vi "NI6071E.evt call Read DAQ.vi"(0 "i ref in":refnum<vi>, 2 "Client":string, 3 "Client timeout (10000)":i32=10000, 4 "NI6071E Read":T1={"time limit in sec (-1:auto calculate)"=1.0, "number of scans to read (-1:all)"=1} {"time limit in sec (-1:auto calculate)" format="%0.2f"}, 5 "error in (no error)":errorcluster) -> (14 "i ref out":refnum<vi>, 16 "error unpacking data":bool, 17 "Data":waveform(dbl)[](array[waveform]), 19 "error out":errorcluster)   [LabVIEW 2014, in "NI6071E.lvlib"]
doc: "This VI asks for an event by a synchronous call"
uses:
  NI6071E.lvlib
  NI6071ECommand.ctl
  NI6071ERead.ctl
  CSCore/CSSystem/CoreLib/CoreLib.string 2 byte array.vi
  CSCore/CSSystem/CoreLib/CoreLib.int 2 byte array.vi
  CSCore/CSSystem/CoreLib/CoreLib.byte array 2 string.vi
  CSCore/BaseProcess/BaseProcess.lvlib
  CSCore/CSSystem/CoreLib/CoreLib.lvlib
panel:
  in  "PreAmp Data 2":waveform(dbl)[](graph) caption="Measurement data"
  in  "NI6071E Command":T2=enum."ReadData"
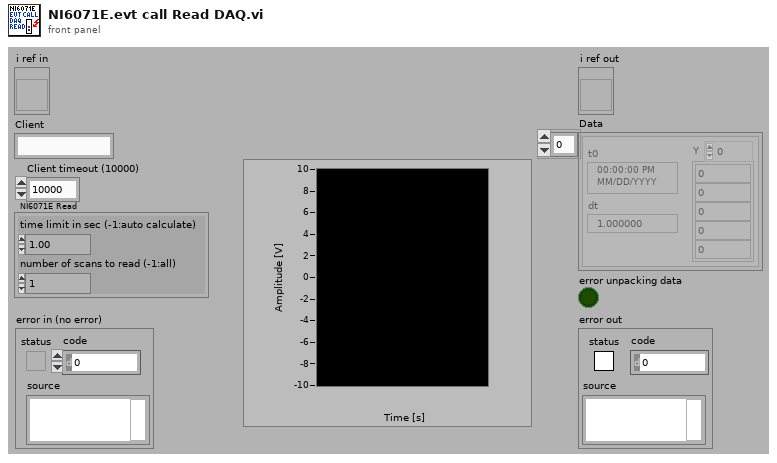
[diagram p1: front panel]
types:
  T1 = typedef "NI6071E.lvlib/NI6071ERead.ctl" = cluster{"time limit in sec (-1:auto calculate)":sgl, "number of scans to read (-1:all)":i32}
  T2 = typedef "NI6071E.lvlib/NI6071ECommand.ctl" = enum16{"Ping", "Reset", "ConfigureDAQ", "StartDAQ", "StopDAQ", "GetDAQStatus", "ReadData", "SaveData", "CloseConnection"}
  T3 = enum16{"simple", "synchronous", "asynchronous", "notification"}
  T4 = typedef "CoreDefs.rawDataType.ctl" = i8[]
  T5 = typedef "CoreDefs.call_type.ctl" = cluster{"Object":string, "Selector":string, "CallType":enum16{"simple", "synchronous", "asynchronous"}, "Async Object":string, "Async Selector":string, "Data Descriptor":T6, "Data":T4, "Error #":i32, "Expire":u32}
  T6 = typedef "BaseProcess.lvlib/BaseProcess.descriptor string definition.ctl" = string
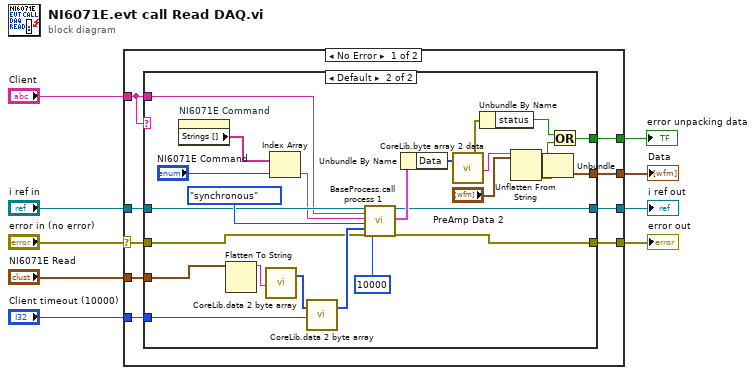
[diagram p0: block diagram]
diagram:
  n1 = case shown="No Error" "error in (no error)" {
    selector: "error in (no error)" -> [w11 w46]
    tunnel: [w18 w46] -> w9
    tunnel: "i ref in" -> [w17 w47]
    tunnel: "Client" -> [w10 _]
    tunnel: [w16 w47] -> w6
    tunnel: "NI6071E Read" -> [w15 _]
    tunnel: [w14 _] -> w4
    tunnel: [w13 _] -> w3
    tunnel: "Client timeout (10000)" -> [w12 _]
    frame No Error {
      n2 = case shown="Default" w10 {
        tunnel: [w19 w44] -> w18
        tunnel: w17 -> [w20 w42]
        tunnel: w10 -> [_ w41]
        tunnel: [w20 w39] -> w16
        tunnel: w15 -> [_ w35]
        tunnel: [_ w33] -> w14
        tunnel: [_ w31] -> w13
        tunnel: w12 -> [_ w23]
        tunnel: w11 -> [w19 w22]
        frame "N/A" {
        }
        frame Default {
          n3 = property on="NI6071E Command" class="Enum (strict)"() -> ("Strings []"=w37:string[])  [unwired: 2 in, 2 out]
          n4 = Flatten To String(anything=w35) -> (data string=w26:string)  [unwired: 3 in, 2 out]
          n5 = call-poly "CoreLib.data 2 byte array.vi"("string"=w26) -> ("byteArray out"=w24:T4)  [unwired: 18 in]
          n6 = Index Array(array=w37, index="NI6071E Command") -> (element=w36:string)
          n7 = call-poly "CoreLib.data 2 byte array.vi"("byteArray"=w24, "i32"=w23) -> ("byteArray out"=w25:T4)  [unwired: 17 in]
          n8 = call "BaseProcess.call process 1.vi"("i ref in"=w42, "Object"=w41, "Selector"=w36, "CallType"=T3."synchronous", "Data"=w25, "error in (no error)"=w22, "timeout (ms)"=10000) -> ("i ref out"=w39:refnum<vi>, "call cluster out"=w45:T5, "error out"=w44:errorcluster)  [unwired: 10 in]
          n9 = Unbundle By Name(w45) -> ("Data"=w30:T4)
          n10 = call-poly "CoreLib.byte array 2 data.vi"("byteArray"=w30) -> ("string"=w29:string, "error out"=w28:errorcluster)  [unwired: 16 in, 1 out]
          n11 = Unbundle By Name(w28) -> ("status"=w27:bool)
          n12 = Unflatten From String(type="PreAmp Data 2", binary string=w29) -> (value=w33:waveform(dbl)[], error out=w21:errorcluster)  [unwired: 3 in, 1 out]
          n13 = Unbundle(w21) -> ("status"=w32:bool)  [unwired: 2 out]
          n14 = Or(x=w27, y=w32) -> (x .or. y?=w31:bool)
        }
      }
    }
    frame Error {
    }
  }
  "error out" <- w9
  "i ref out" <- w6
  "Data" <- w4
  "error unpacking data" <- w3
